vi "main2.3.vi"() -> ()   [LabVIEW 2023]
uses:
  <extravilib>/ChannelInstances/Tag-path/Read With Abort.vi
  <extravilib>/ChannelInstances/Tag-a[.](wfm(dbl))/Read With Abort.vi
  <extravilib>/ChannelInstances/Tag-c(bool,i32,str)/Read With Abort.vi
  <extravilib>/ChannelInstances/Tag-bool/Read With Abort.vi
  <extravilib>/ChannelInstances/Tag-path/Write With Abort.vi
  <extravilib>/ChannelInstances/Tag-c(bool,i32,str)/Write With Abort.vi
  <extravilib>/ChannelInstances/Tag-bool/Write With Abort.vi
  <extravilib>/ChannelInstances/Tag-a[.](wfm(dbl))/Write With Abort.vi
  <extravilib>/ChannelInstances/Tag-path/Instantiate.vi
  <extravilib>/ChannelInstances/Tag-a[.](wfm(dbl))/Instantiate.vi
  <extravilib>/ChannelInstances/Tag-c(bool,i32,str)/Instantiate.vi
  <extravilib>/ChannelInstances/Tag-bool/Instantiate.vi
  <extravilib>/ChannelInstances/Tag-path/EndpointRead.vi
  <extravilib>/ChannelInstances/Tag-a[.](wfm(dbl))/EndpointRead.vi
  <vilib>/express/express shared/transition.llb/Dynamic To Waveform Array.vi
  <vilib>/express/express signal manip/GetorSetDDTAttributes/Set DDT Attributes/SetT0.vi
  <vilib>/express/express shared/transition.llb/Waveform Array To Dynamic.vi
  <extravilib>/ChannelInstances/Tag-c(bool,i32,str)/EndpointRead.vi
  <extravilib>/ChannelInstances/Tag-bool/EndpointRead.vi
  <extravilib>/ChannelInstances/Tag-path/Endpoint.vi
  <extravilib>/ChannelInstances/Tag-c(bool,i32,str)/Endpoint.vi
  <extravilib>/ChannelInstances/Tag-bool/Endpoint.vi
  <extravilib>/ChannelInstances/Tag-a[.](wfm(dbl))/Endpoint.vi
  <vilib>/express/express signal manip/GetorSetDDTAttributes/Set DDT Attributes/Set DDT Properties.xnode
  <vilib>/MakerHub/Toolbox/LMH-Toolbox.lvlib
  <extravilib>/ChannelInstances/Tag-bool.lvlib
  <extravilib>/ChannelInstances/Tag-c(bool,i32,str).lvlib
  <extravilib>/ChannelInstances/Tag-path.lvlib
  <extravilib>/ChannelInstances/Tag-a[.](wfm(dbl)).lvlib
panel:
  out "Time(Sec)":i32
  out "Current Calibration":dbl[](array[numeric])
  in  "Calibration":dbl[](array[numeric])
  out "a 2":dbl[](array[numeric])
  out "a":dbl[](array[numeric])
  out "Ch Temps °F":dbl[](array[numeric])
  out "Numeric":i32
  out "File Location":string
  in  "File  Name":string
  in  "Save":bool
  out "Thermistor Unfiltered 2":waveform(dbl)[](graph)
  out "XY Graph":cluster{timestamp[], "Y":dbl[]}[](graph)
  out "Thermistor Filtered":T1(graph)
  out "Thermistor Unfiltered":T2(graph)
  in  "Thermistor":T3
  out "Waveform Chart 3":T4(graph)
  in  "error in (no error)":errorcluster
  out "error out":errorcluster
  out "Waveform Chart 2":waveform(dbl)(graph)
  out "a0 Scalar Voltage":dbl
  out "Waveform Chart":dynamicdata(graph)
  in  "stop":bool
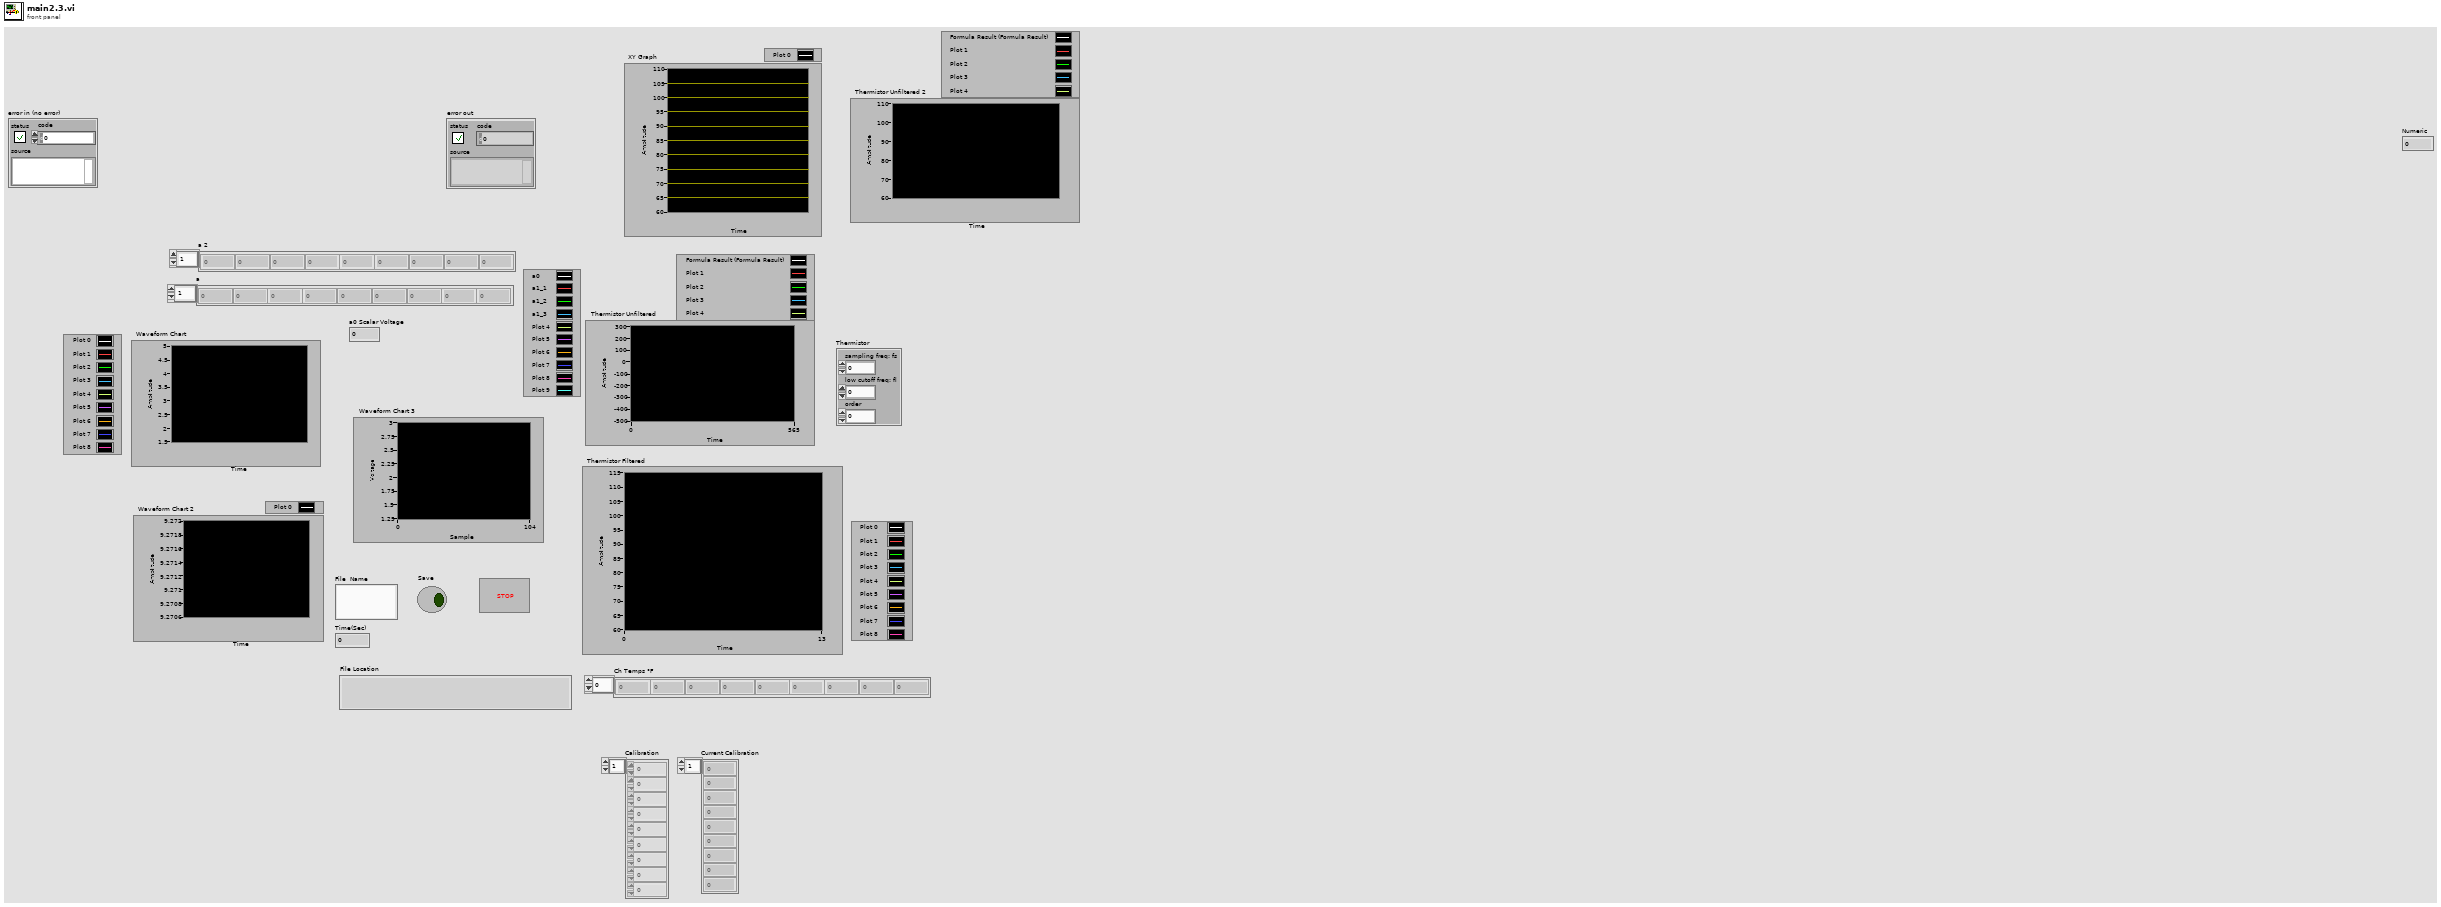
[diagram p1: front panel]
types:
  T1 = cluster{"Temp Filtered[0]":dbl, "Temp Filtered[1]":dbl, "Temp Filtered[2]":dbl, "Temp Filtered[3]":dbl, "Temp Filtered[4]":dbl, "Temp Filtered[5]":dbl, "Temp Filtered[6]":dbl, "Temp Filtered[7]":dbl, "Temp Filtered[8]":dbl}
  T2 = cluster{"[0]":dbl, "[1]":dbl, "[2]":dbl, "[3]":dbl, "[4]":dbl, "[5]":dbl, "[6]":dbl, "[7]":dbl, "[8]":dbl}
  T3 = cluster{"sampling freq: fs":dbl, "low cutoff freq: fl":dbl, "order":i32}
  T4 = cluster{"Data_Array[0]":dbl, "Data_Array[1]":dbl, "Data_Array[2]":dbl, "Data_Array[3]":dbl, "Data_Array[4]":dbl, "Data_Array[5]":dbl, "Data_Array[6]":dbl, "Data_Array[7]":dbl, "Data_Array[8]":dbl}
  T5 = cluster{"Data_Array":dbl[], "Multiplex_Tbl":u32[]}
  T6 = cluster{"Temp[0]":dbl, "Temp[1]":dbl, "Temp[2]":dbl, "Temp[3]":dbl, "Temp[4]":dbl, "Temp[5]":dbl, "Temp[6]":dbl, "Temp[7]":dbl, "Temp[8]":dbl}
  T7 = typedef "Tag-path.lvlib/))Channel.ctl" = refnum<queue>
  T8 = typedef "Tag-a[.](wfm(dbl)).lvlib/))Channel.ctl" = refnum<queue>
  T9 = typedef "Tag-bool.lvlib/))Channel.ctl" = refnum<queue>
  T10 = typedef "Tag-c(bool,i32,str).lvlib/))Channel.ctl" = refnum<queue>
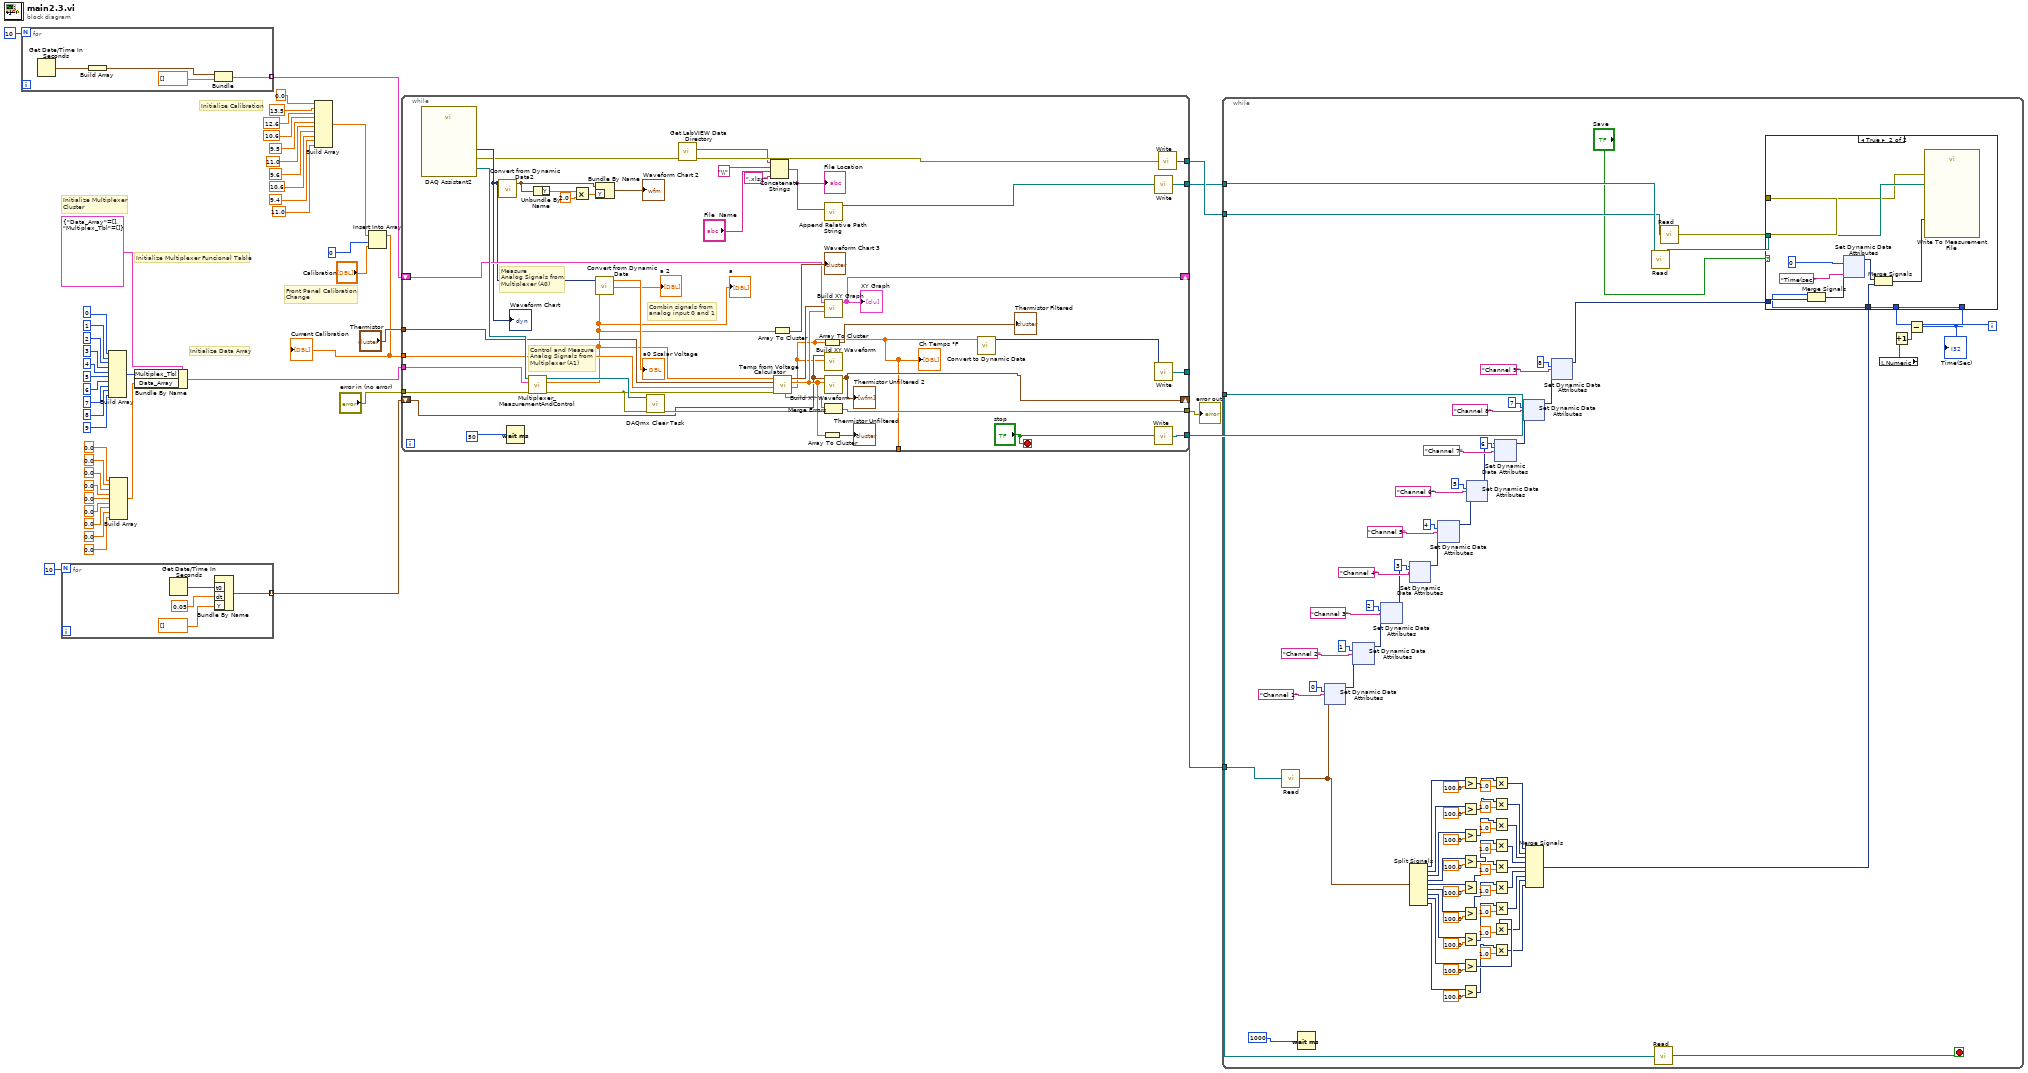
[diagram p0: block diagram]
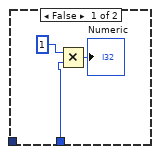
[diagram p2: hidden frame]
diagram:
  # "Front Panel Calibration\nChange"
  # "Initialize Calibration"
  # "Initialize Multiplexer \nCluster"
  # "Initialize Data Array"
  # "Initialize Multiplexer Funcional Table"
  n1 = for {
    N: 10 -> [_]
    tunnel: [w50] -> w37 mode=indexing
    n2 = Get Date/Time In Seconds() -> (seconds since 1Jan1904=w52:timestamp)
    n3 = Build Array(w52) -> (w51:timestamp[])
    n4 = Bundle(w51, "Y"=dbl[] []) -> (w50:cluster{timestamp[], "Y":dbl[]})  [unwired: 1 in]
  }
  n5 = for {
    N: 10 -> [_]
    tunnel: [w53] -> w34 mode=indexing
    n6 = Get Date/Time In Seconds() -> (seconds since 1Jan1904=w55:timestamp)
    n7 = Bundle By Name("t0"=w55, "dt"=0.05, "Y"=dbl[] []) -> (w53:waveform(dbl))  [unwired: 1 in]
  }
  n8 = Build Array(0, 1 ("Waveform"), u32 2 ("Waveform"), 3, 4, 5, 6, 7, 8, 9) -> (w39:u32[])
  n9 = Build Array(0.0 ("element"), 0.0 ("element"), 0.0 ("element"), 0.0, 0.0, 0.0, 0.0, 0.0, 0.0) -> (w44:dbl[])
  n10 = Bundle By Name(cluster=T5 {"Data_Array"=[], "Multiplex_Tbl"=[]}, "Multiplex_Tbl"=w39, "Data_Array"=w44) -> (w43:T5)
  n11 = Build Array(0.0, 13.5 ("element"), 12.6 ("element"), 10.6 ("element"), 9.5, 11.0, 9.6, 10.6, 9.4, 11.0) -> (w3:dbl[])
  n12 = Insert Into Array(array=w3, index=0, new element="Calibration") -> (w6:dbl[])
  "Current Calibration" <- w6
  n13 = while {
    tunnel: w43 -> [w93]
    tunnel: "error in (no error)" -> [w92]
    tunnel: "Thermistor" -> [w87]
    shift-right: [w84] -> _
    shift-left: w37 -> [w85]
    shift-right: [w62] -> _
    shift-left: w34 -> [w78]
    tunnel: w6 -> [w79]
    tunnel: [w77] -> w30
    tunnel: [w68] -> w10
    tunnel: [w67] -> w9
    tunnel: [w66] -> w7
    tunnel: [w65] -> w8
    tunnel: [w59] -> _
    stop <- "stop" stop-if-true
    # "Combin signals from \nanalog input 0 and 1"
    # "Measure\nAnalog Signals from\nMultiplexer (A0)"
    # "Control and Measure\nAnalog Signals from\nMultiplexer (A1)"
    n14 = call "DAQ Assistant2"() -> ("task out"=w91:refnum<k21>, "data"=w76:dynamicdata, "error out"=w74:errorcluster)  [unwired: 16 in, 1 out]
    "Waveform Chart" <- w76
    n15 = call "Convert from Dynamic Data2"("Dynamic Data Type"=w76) -> ("Waveform"=w96:waveform(dbl))  [unwired: 3 in]
    n16 = Wait (ms)(milliseconds to wait=50) -> ()  [unwired: 1 out]
    n17 = call "Multiplexer_MeasurementAndControl.vi"("error in (no error)"=w92, "Multiplexer_Cluser"=w93, "Task in"=w91) -> ("error out"=w82:errorcluster, "Data_Array"=w60:dbl[], "Task out"=w88:refnum<k21>)  [unwired: 6 in]
    "a" <- w60
    "a 2" <- w60
    n18 = Unbundle By Name(w96) -> ("Y"=w98:dbl[])
    n19 = Multiply(x=w98, y=2.0) -> (x*y=w95:dbl[])
    n20 = Bundle By Name(cluster=w96, "Y"=w95) -> (→"Waveform Chart 2":waveform(dbl))
    n21 = call "Convert from Dynamic Data"("Dynamic Data Type"=w76) -> ("Scalar"=→"a0 Scalar Voltage":dbl)  [unwired: 3 in]
    n22 = call <vilib>:"DAQmx Clear Task.vi"("task in"=w88, "error in"=w82) -> ("error out"=w81:errorcluster)  [unwired: 13 in]
    n23 = call <vilib>:"Get LabVIEW Data Directory.vi"("Error In"=w74) -> ("Error Out"=w69:errorcluster, "LabVIEW Data Path"=w58:string)  [unwired: 9 in]
    n24 = Concatenate Strings(w58, "\\", "File  Name", ".xlsx") -> (w71:string)
    "File Location" <- w71
    n25 = Array To Cluster(array=w60) -> (cluster=→"Waveform Chart 3":T4)
    n26 = call "Temp from Voltage Calculator.vi"("error in (no error)"=w82, "Calibrations"=w79, "Thermistor"=w87, "Data_Array"=w60) -> ("Temp Filtered"=w59:dbl[], "Temp"=w83:dbl[], "Time Read"=w80:timestamp[], "error out"=w75:errorcluster[])  [unwired: 4 in]
    "Ch Temps °F" <- w59
    n27 = Array To Cluster(array=w59) -> (cluster=→"Thermistor Filtered":T1)
    n28 = Array To Cluster(array=w83) -> (cluster=→"Thermistor Unfiltered":T6)
    n29 = call <vilib>:"Append Relative Path String.vi"("Relative Path"=w71) -> ("Absolute Path"=w70:path)  [unwired: 9 in, 1 out]
    n30 = call "Build XY Graph.vi"("Meas Temp"=w83, "Meas Time"=w80, "XY In"=w85) -> ("XY out"=w84:cluster{timestamp[], "Y":dbl[]}[])  [unwired: 8 in]
    "XY Graph" <- w84
    n31 = call "Build XY Waveform.vi"("New Temps"=w59, "Waveforms in"=w78) -> ()  [unwired: 9 in, 1 out]
    n32 = call "Build XY Waveform.vi"("New Temps"=w83, "Waveforms in"=w78) -> ("Waveforms out"=w62:waveform(dbl)[])  [unwired: 9 in]
    "Thermistor Unfiltered 2" <- w62
    n33 = Merge Errors(w75, w81) -> (w77:errorcluster)
    n34 = call "Convert to Dynamic Data"("Array"=w59) -> ("Dynamic Data Type"=w61:dynamicdata)  [unwired: 3 in]
    n35 = call <extravilib>:"Write.vi"("element"=w70) -> ("channel"=w66:T7)  [unwired: 1 out]
    n36 = call <extravilib>:"Write.vi"("element"=w61) -> ("channel"=w65:T8)  [unwired: 1 out]
    n37 = call <extravilib>:"Write.vi"("element"="stop") -> ("channel"=w68:T9)  [unwired: 1 out]
    n38 = call <extravilib>:"Write.vi"("element"=w69) -> ("channel"=w67:T10)  [unwired: 1 out]
  }
  "error out" <- w30
  n39 = while {
    tunnel: w10 -> [w186]
    tunnel: w9 -> [w159]
    tunnel: w8 -> [w161]
    tunnel: w7 -> [w160]
    i -> [w158]
    stop <- w185 stop-if-true
    n40 = call <extravilib>:"Read.vi"("channel"=w161) -> ("element"=w147:waveform(dbl)[])  [unwired: 1 in, 1 out]
    n41 = Wait (ms)(milliseconds to wait=1000) -> ()  [unwired: 1 out]
    n42 = xnode "Set Dynamic Data Attributes"("Signals In"=w147, "Signal Index"=0, "Signal Name"="Channel 1") -> ("Signals Out"=w156:dynamicdata)  [unwired: 1 in, 1 out]
    n43 = xnode "Set Dynamic Data Attributes"("Signals In"=w156, "Signal Index"=1, "Signal Name"="Channel 2") -> ("Signals Out"=w155:dynamicdata)  [unwired: 1 in, 1 out]
    n44 = xnode "Set Dynamic Data Attributes"("Signals In"=w155, "Signal Index"=2, "Signal Name"="Channel 3") -> ("Signals Out"=w154:dynamicdata)  [unwired: 1 in, 1 out]
    n45 = xnode "Set Dynamic Data Attributes"("Signals In"=w154, "Signal Index"=3, "Signal Name"="Channel 4") -> ("Signals Out"=w153:dynamicdata)  [unwired: 1 in, 1 out]
    n46 = Split Signals(w147) -> (w146:dynamicdata, w143:dynamicdata, w141:dynamicdata, w139:dynamicdata, w137:dynamicdata, w135:dynamicdata, w133:dynamicdata, w131:dynamicdata, w129:dynamicdata)  [unwired: 9 in]
    n47 = xnode "Set Dynamic Data Attributes"("Signals In"=w153, "Signal Index"=4, "Signal Name"="Channel 5") -> ("Signals Out"=w152:dynamicdata)  [unwired: 1 in, 1 out]
    n48 = Greater?(x=w146, y=100.0) -> (0:w128:dynamicdata)
    n49 = Greater?(x=w143, y=100.0) -> (0:w125:dynamicdata)
    n50 = Greater?(x=w141, y=100.0) -> (0:w123:dynamicdata)
    n51 = Greater?(x=w139, y=100.0) -> (0:w121:dynamicdata)
    n52 = Greater?(x=w137, y=100.0) -> (0:w119:dynamicdata)
    n53 = Greater?(x=w135, y=100.0) -> (0:w117:dynamicdata)
    n54 = Greater?(x=w133, y=100.0) -> (0:w115:dynamicdata)
    n55 = Greater?(x=w131, y=100.0) -> (0:w113:dynamicdata)
    n56 = Greater?(x=w129, y=100.0) -> (0:w111:dynamicdata)
    n57 = xnode "Set Dynamic Data Attributes"("Signals In"=w152, "Signal Index"=5, "Signal Name"="Channel 6") -> ("Signals Out"=w151:dynamicdata)  [unwired: 1 in, 1 out]
    n58 = Multiply(x=w128, y=1.0) -> (x*y=w110:dynamicdata)
    n59 = Multiply(x=w125, y=1.0) -> (x*y=w109:dynamicdata)
    n60 = Multiply(x=w123, y=1.0) -> (x*y=w108:dynamicdata)
    n61 = Multiply(x=w121, y=1.0) -> (x*y=w107:dynamicdata)
    n62 = Multiply(x=w119, y=1.0) -> (x*y=w106:dynamicdata)
    n63 = Multiply(x=w117, y=1.0) -> (x*y=w105:dynamicdata)
    n64 = Multiply(x=w115, y=1.0) -> (x*y=w104:dynamicdata)
    n65 = Multiply(x=w113, y=1.0) -> (x*y=w103:dynamicdata)
    n66 = Multiply(x=w111, y=1.0) -> (x*y=w102:dynamicdata)
    n67 = xnode "Set Dynamic Data Attributes"("Signals In"=w151, "Signal Index"=6, "Signal Name"="Channel 7") -> ("Signals Out"=w150:dynamicdata)  [unwired: 1 in, 1 out]
    n68 = xnode "Set Dynamic Data Attributes"("Signals In"=w150, "Signal Index"=7, "Signal Name"="Channel 8") -> ("Signals Out"=w149:dynamicdata)  [unwired: 1 in, 1 out]
    n69 = Merge Signals(w110, w109, w108, w107, w106, w105, w104, w103, w102) -> (w100:dynamicdata)
    n70 = xnode "Set Dynamic Data Attributes"("Signals In"=w149, "Signal Index"=8, "Signal Name"="Channel 9") -> ("Signals Out"=w183:dynamicdata)  [unwired: 1 in, 1 out]
    n71 = call <extravilib>:"Read.vi"("channel"=w160) -> ("element"=w101:path)  [unwired: 1 in, 1 out]
    n72 = call <extravilib>:"Read.vi"("channel"=w186) -> ("element"=w185:bool)  [unwired: 1 in, 1 out]
    n73 = call <extravilib>:"Read.vi"("channel"=w159) -> ("element"=w180:errorcluster)  [unwired: 1 in, 1 out]
    n74 = local read "Numeric"() -> (w181:i32)
    n75 = Increment(x=w181) -> (x+1=w182:i32)
    n76 = Subtract(x=w158, y=w182) -> (x-y=w148:i32)
    "Time(Sec)" <- w148
    n77 = case shown="True" "Save" {
      tunnel: w101 -> [_ w316]
      tunnel: w180 -> [_ w315]
      tunnel: w183 -> [_ w314]
      tunnel: w158 -> [w306 _]
      tunnel: w148 -> [_ w313]
      tunnel: w100 -> [_ w309]
      frame False {
        n78 = Multiply(x=1, y=w306) -> (x*y=→"Numeric":i32)
      }
      frame True {
        n79 = Merge Signals(w313, w314) -> (w310:dynamicdata)
        n80 = xnode "Set Dynamic Data Attributes"("Signals In"=w310, "Signal Index"=0, "Signal Name"="Time(sec)") -> ("Signals Out"=w308:dynamicdata)  [unwired: 1 in, 1 out]
        n81 = Merge Signals(w308, w309) -> (w307:dynamicdata)
        n82 = call "Write To Measurement File"("Signals"=w307, "error in (no error)"=w315, "Filename"=w316) -> ()  [unwired: 14 in, 3 out]
      }
    }
  }
